vi "Untitled 1 (SubVI).vi"(11 "read buffer":string) -> (3 "Numeric":dbl)   [LabVIEW 2024]
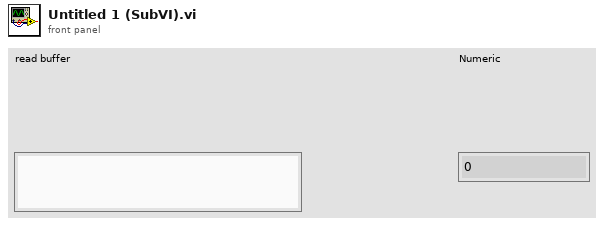
[diagram p1: front panel]
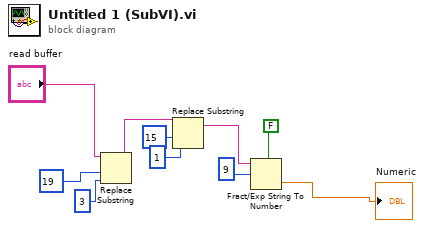
[diagram p0: block diagram]
diagram:
  n1 = Replace Substring(2:3 ("length (len. of substring)"), 3:19 ("offset (0)"), 5:"read buffer") -> (1:w7:string)  [unwired: 1 in, 1 out]
  n2 = Replace Substring(2:1 ("length (len. of substring)"), 3:15 ("offset (0)"), 5:w7) -> (1:w10:string)  [unwired: 1 in, 1 out]
  n3 = Fract/Exp String To Number(use system decimal point (T)=FALSE, string=w10, offset=9) -> (number=→"Numeric":dbl)  [unwired: 1 in, 1 out]
